vi "Import_Old_Text.vi"(1 "Input Text":string[](array[string])) -> (0 "Output Text":string[](array[string]))   [LabVIEW 2011]
doc: "This VI fixes several problems in older text sequences that prevent correct parsing."
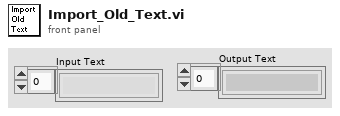
[diagram p1: front panel]
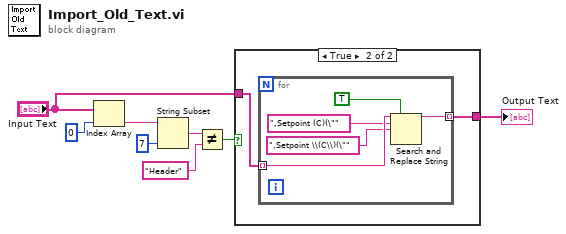
[diagram p0: block diagram]
diagram:
  n1 = Index Array(array="Input Text", index=0) -> (element=w8:string)
  n2 = String Subset(string=w8, length (rest)=7 ("length (rest)")) -> (substring=w6:string)  [unwired: 1 in]
  n3 = Not Equal?(x=w6, y="Header") -> (x != y?=w4:bool)
  n4 = case shown="True" w4 {
    tunnel: [_ w10] -> w3
    tunnel: "Input Text" -> [_ w9]
    frame False {
    }
    frame True {
      n5 = for {
        tunnel: w9 -> [w15] mode=indexing
        tunnel: [w11] -> w10 mode=indexing
        n6 = Search and Replace String(replace all?=TRUE ("replace all? (F)"), input string=w15, search string=",Setpoint (C)(\"" ("input string"), replace string=",Setpoint \\(C\\)(\"" ("replace string (\"\")")) -> (result string=w11:string)  [unwired: 4 in, 3 out]
      }
    }
  }
  "Output Text" <- w3
